vi "loadFile.vi"(11 "file path (dialog if empty)":path) -> (2 "B-Cave":dbl[](array[numeric]), 3 "A-Cave":dbl[](array[numeric]))   [LabVIEW 2013]
uses:
  <vilib>/Utility/file.llb/Read From Spreadsheet File (string).vi
panel:
  out "array w/ subset deleted 2":string[](array[string])
  out "all rows":string[][](array[string])
  out "array w/ subset deleted":string[][](array[string])
  out "deleted portion":string[](array[string])
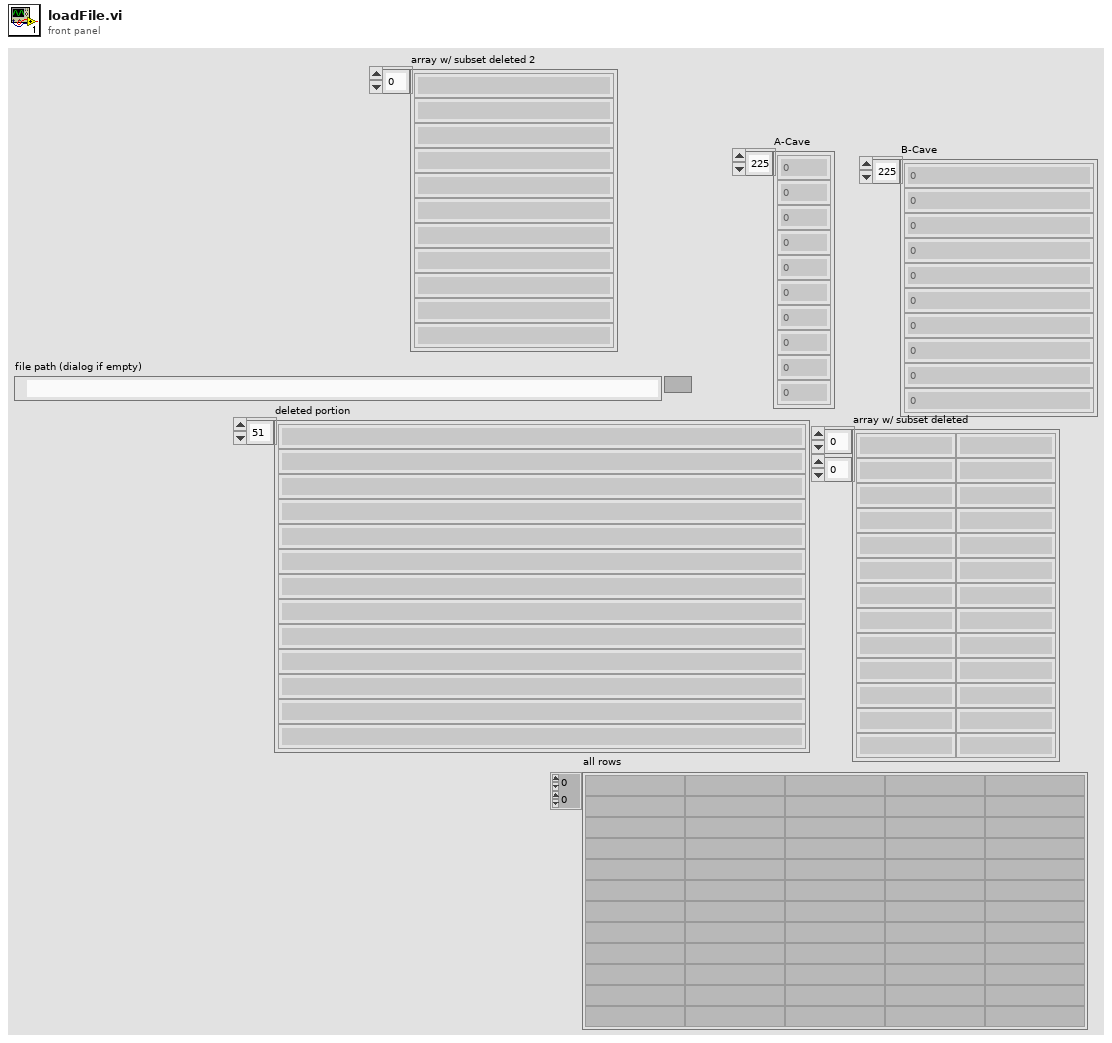
[diagram p1: front panel]
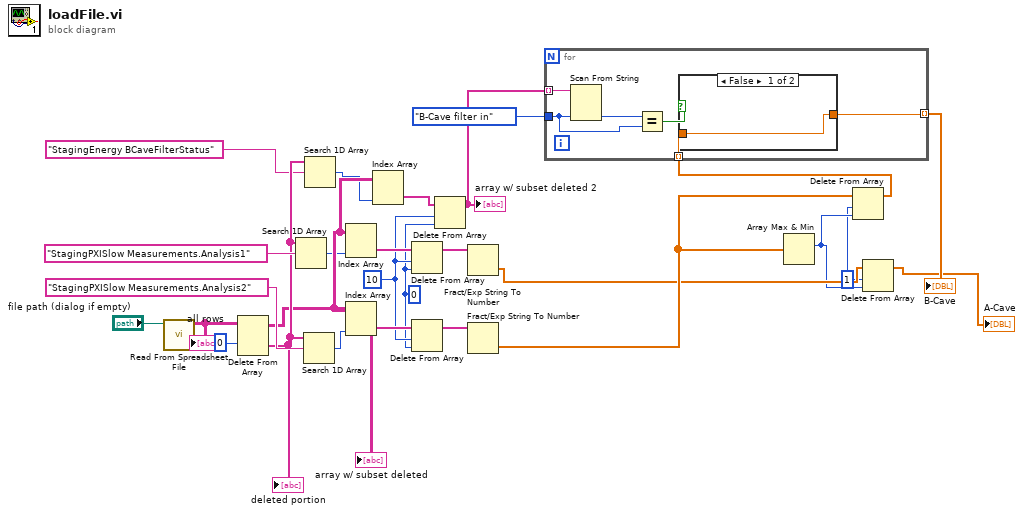
[diagram p0: block diagram]
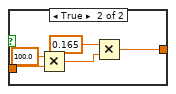
[diagram p2: hidden frame]
diagram:
  w3 = 1 ("length")
  w11 = 0 ("index")
  w12 = 10 ("length")
  n1 = call-poly <vilib>:"Read From Spreadsheet File.vi"("file path (dialog if empty)"="file path (dialog if empty)") -> ("all rows"=w26:string[][])  [unwired: 6 in, 4 out]
  "all rows" <- w26
  n2 = Delete From Array(array=w26, index (row)=0) -> (deleted portion=w17:string[], array with subset deleted=w15:string[][])  [unwired: 2 in]
  "deleted portion" <- w17
  "array w/ subset deleted" <- w15
  n3 = Search 1D Array(1D array=w17, element="StagingPXISlow Measurements.Analysis1") -> (index of element=w14:i32)  [unwired: 1 in]
  n4 = Search 1D Array(1D array=w17, element="StagingPXISlow Measurements.Analysis2") -> (index of element=w22:i32)  [unwired: 1 in]
  n5 = Search 1D Array(1D array=w17, element="StagingEnergy BCaveFilterStatus") -> (index of element=w10:i32)  [unwired: 1 in]
  n6 = Index Array(array=w15, index (col)=w14) -> (element=w20:string[])  [unwired: 1 in]
  n7 = Index Array(array=w15, index (col)=w22) -> (element=w21:string[])  [unwired: 1 in]
  n8 = Index Array(array=w15, index (col)=w10) -> (element=w13:string[])  [unwired: 1 in]
  n9 = Delete From Array(array=w20, length=w12, index=w11) -> (array with subset deleted=w19:string[])  [unwired: 1 out]
  n10 = Delete From Array(array=w21, length=w12, index=w11) -> (array with subset deleted=w18:string[])  [unwired: 1 out]
  n11 = Delete From Array(array=w13, length=w12, index=w11) -> (array with subset deleted=w9:string[])  [unwired: 1 out]
  "array w/ subset deleted 2" <- w9
  n12 = Fract/Exp String To Number(string=w19) -> (number=w5:dbl[])  [unwired: 3 in, 1 out]
  n13 = Fract/Exp String To Number(string=w18) -> (number=w6:dbl[])  [unwired: 3 in, 1 out]
  n14 = Array Max & Min(array=w6) -> (max index (indices)=w4:i32)  [unwired: 3 out]
  n15 = Delete From Array(array=w6, length=w3, index=w4) -> (array with subset deleted=w2:dbl[])  [unwired: 1 out]
  n16 = for {
    tunnel: w9 -> [w33] mode=indexing
    tunnel: enum16{"B-Cave filter in", "B-Cave filter out"}."B-Cave filter in" ("BCaveFilterStatus") -> [w31]
    tunnel: w2 -> [w29] mode=indexing
    tunnel: [w28] -> w7 mode=indexing
    n17 = Scan From String(input string=w33, default 1=w31) -> (output 1=w32:enum16{"B-Cave filter in", "B-Cave filter out"})  [unwired: 3 in, 3 out]
    n18 = Equal?(x=w32, y=w31) -> (x = y?=w30:bool)
    n19 = case shown="False" w30 {
      tunnel: w29 -> [w34 w39]
      tunnel: [w34 w35] -> w28
      frame False {
      }
      frame True {
        n20 = Multiply(x=100.0, y=w39) -> (x*y=w36:dbl)
        n21 = Multiply(x=0.165, y=w36) -> (x*y=w35:dbl)
      }
    }
  }
  "B-Cave" <- w7
  n22 = Delete From Array(array=w5, length=w3, index=w4) -> (array with subset deleted=→"A-Cave":dbl[])  [unwired: 1 out]
